vi "spannung-akku.vi"(11 "Dynamic Data in":dynamicdata(waveform)) -> (3 "Dynamic Data out":dynamicdata(waveform))   [LabVIEW 2018]
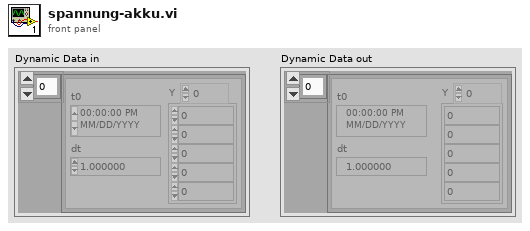
[diagram p1: front panel]
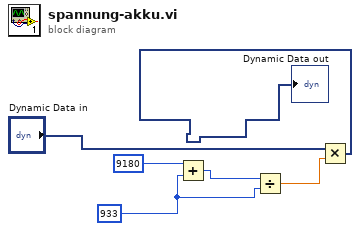
[diagram p0: block diagram]
diagram:
  w4 = 933
  n1 = Add(x=9180, y=w4) -> (x+y=w3:i32)
  n2 = Divide(x=w3, y=w4) -> (x/y=w5:dbl)
  n3 = Multiply(x="Dynamic Data in", y=w5) -> (x*y=→"Dynamic Data out":dynamicdata)
